vi "test Datatype Conversion.vi"(8 "error in (no error)":errorcluster, 11 "TestCase in":refnum<class "SLSC EDS Unit Tests.lvclass">) -> (0 "error out":errorcluster, 3 "TestCase out":refnum<class "SLSC EDS Unit Tests.lvclass">)   [LabVIEW 2015, in "SLSC EDS Unit Tests.lvclass"]
uses:
  SLSC EDS Unit Tests.lvclass
  <vilib>/Utility/Data Type/Type Definitions/Data Type.ctl
  <vilib>/addons/_JKI Toolkits/VI Tester/TestCase.llb/TestCase.lvclass
  <vilib>/Utility/Data Type/NI_Data Type.lvlib
  SLSC UI API/SLSC Tree Control.lvlib
panel:
  out "Pass?":bool
  out "U64":u64
  out "I32":i32
  out "I8":i8
  out "I64":i64
  out "Reset Variant Check":bool[](array[boolean])
  out "Reset = Value?":bool[](array[boolean])
  out "Value Variant Check":bool[](array[boolean])
  out "String Comparison":bool[](array[boolean])
  out "NewVal":variant
  out "Value 2 (DBL)":dbl format="%#_16f"
  out "Value":variant
  out "string data value":string
  out "Type":T1
  out "Value (DBL)":dbl format="%#_16f"
  out "U64 2":u64
  out "Numeric":i32
  in  "Ring":u16(ring)
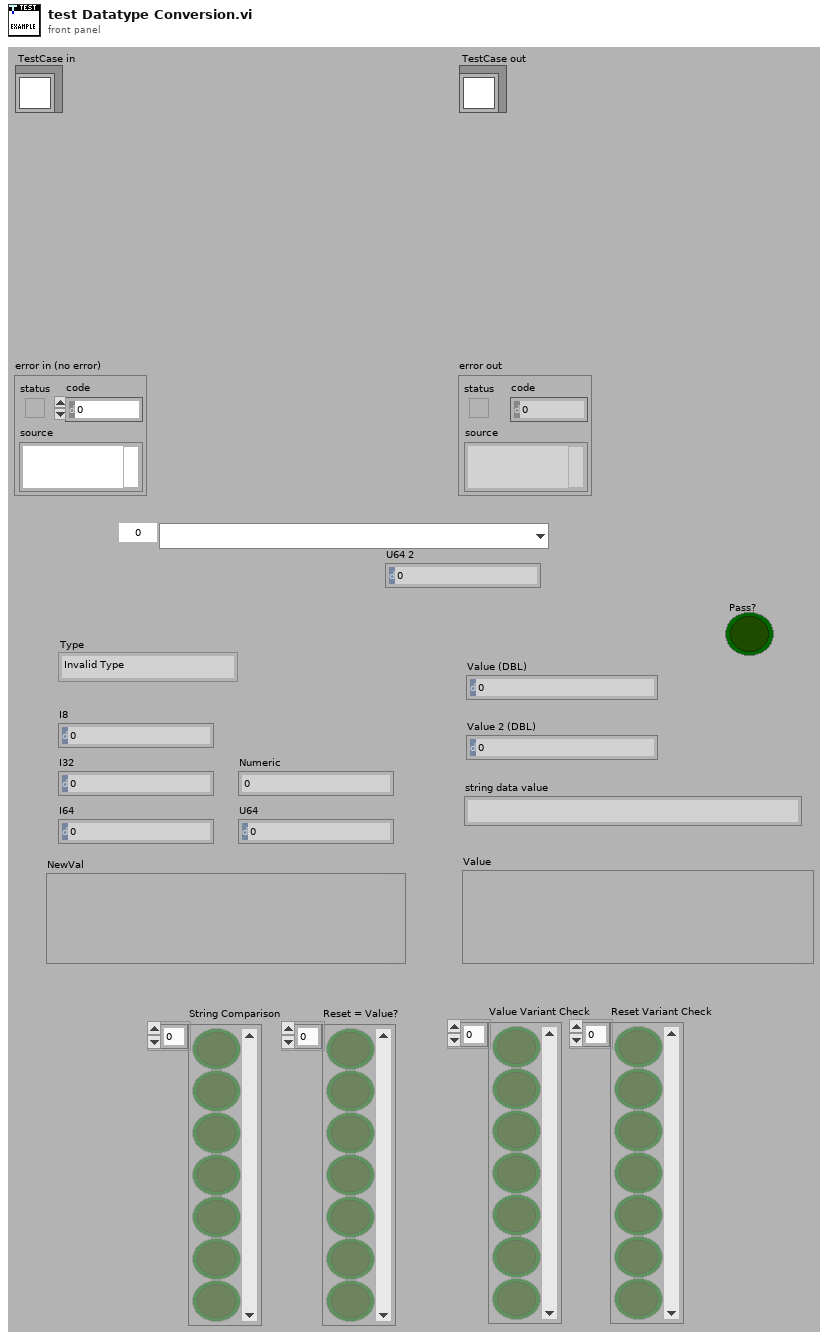
[diagram p1: front panel]
types:
  T1 = typedef "NI_Data Type.lvlib/Data Type.ctl" = enum8{"Invalid Type", "Void", "I8", "I16", "I32", "I64", "U8", "U16", "U32", "U64", "Single Float", "Double Float", "Extended Float", "Single Complex", "Double Complex", "Extended Complex", "Enum U8", "Enum U16", "Enum U32", "Enum U64", "Single Float With Unit", "Double Float With Unit", "Extended Float With Unit", "Single Complex with Unit", "Double Complex with Unit", "Extended Complex with Unit", "Boolean", "String", "Path", "Picture", "Tag", "Array", "Cluster", "Variant", "LV Variant", "Waveform", "Timestamp", "Digital Waveform", "Digital Data", "ExpressData", "Refnum", "External Data", "VI", "Poly VI", "LabVIEW Class Instance", "Fixed Point"}
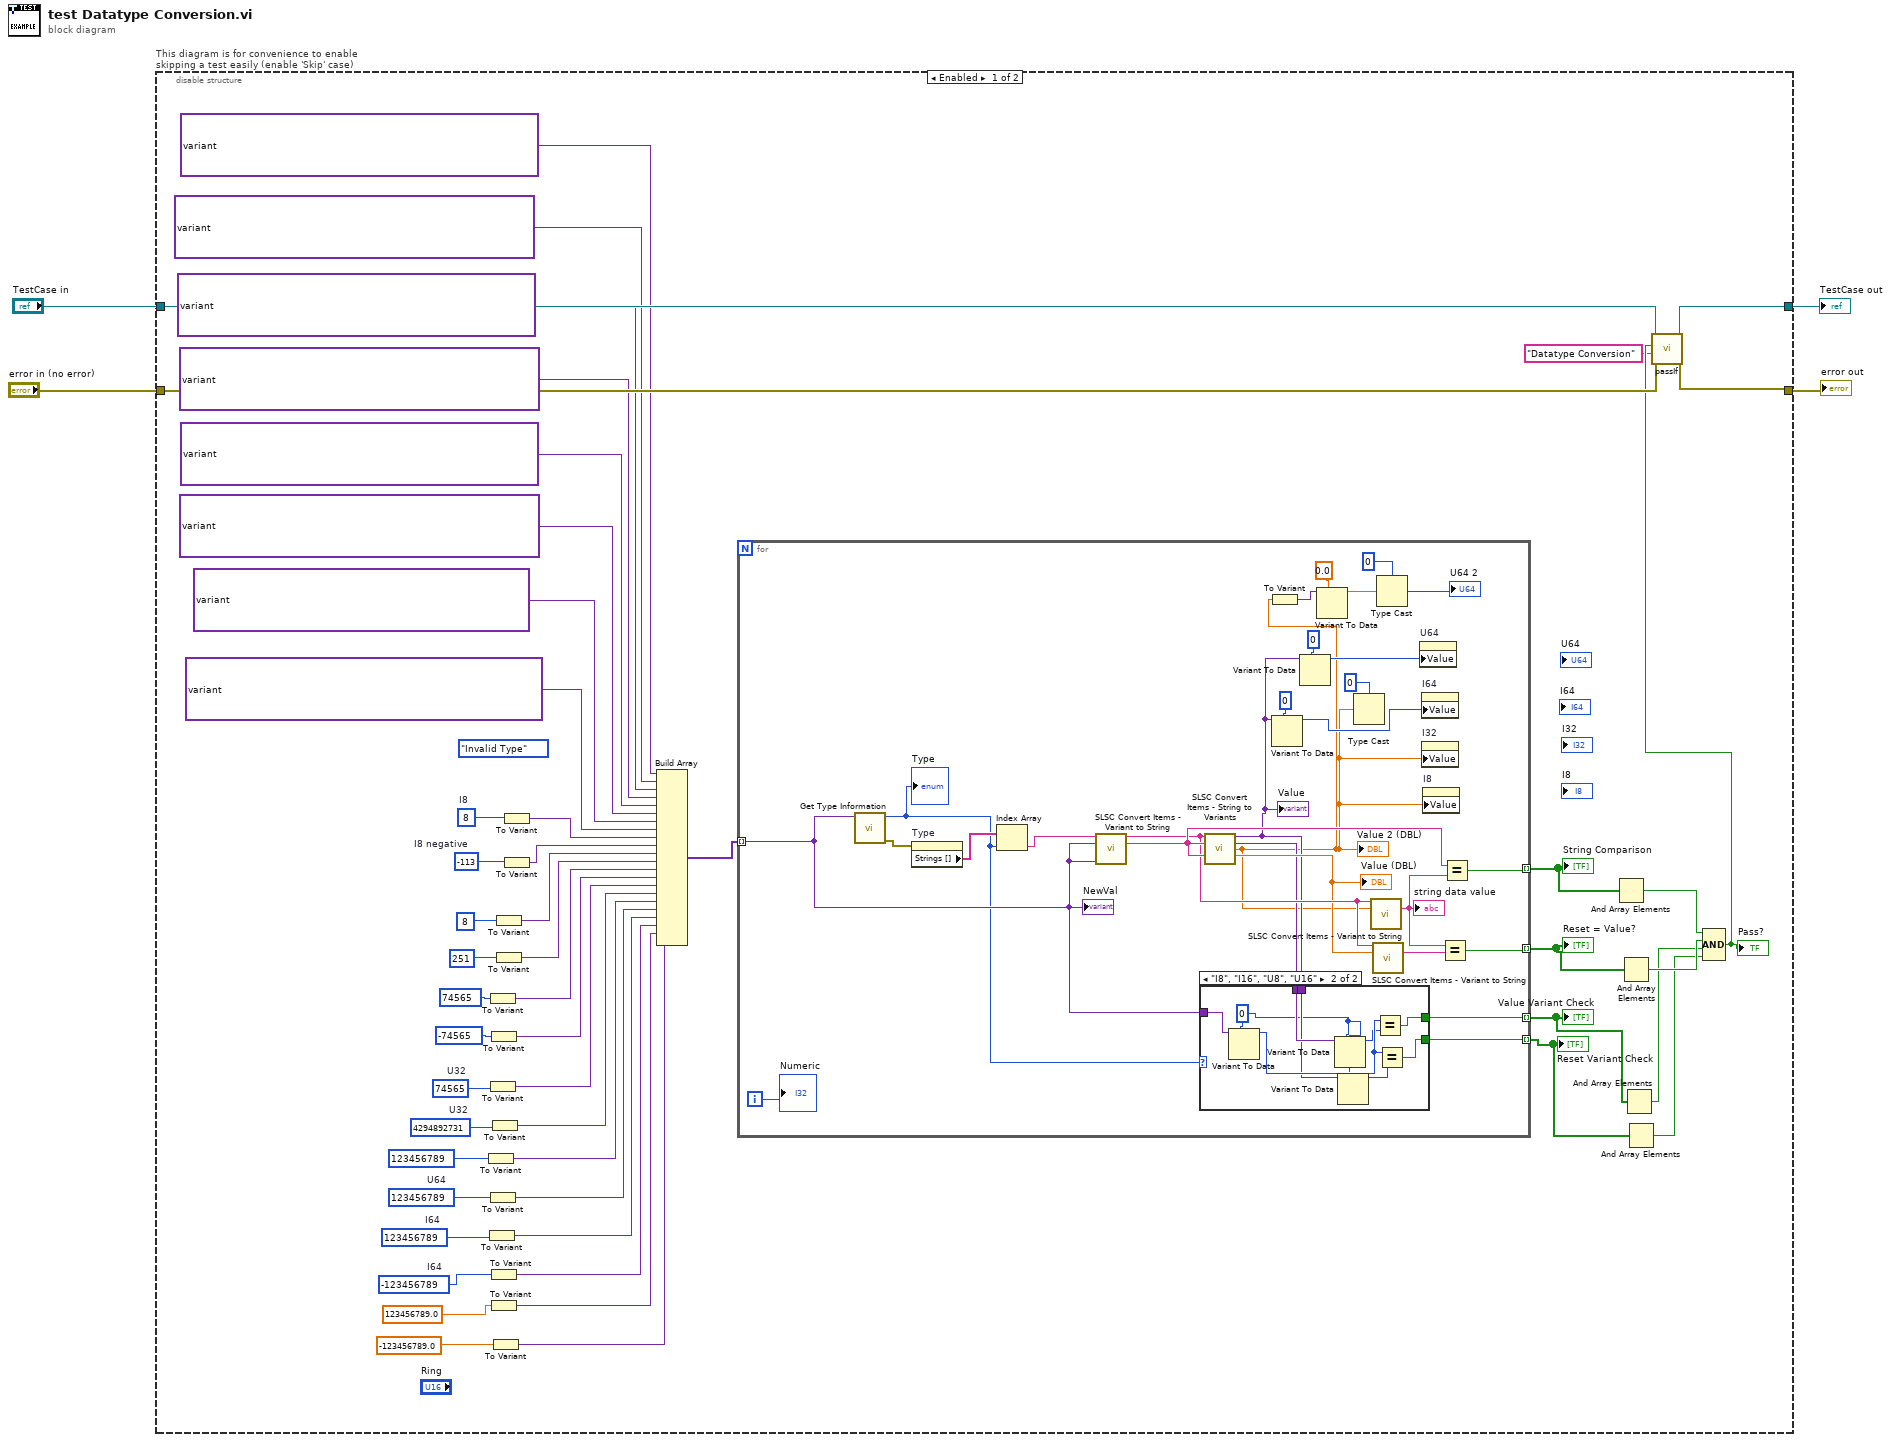
[diagram p0: block diagram]
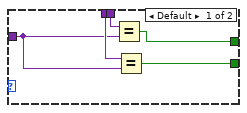
[diagram p2: hidden frame]
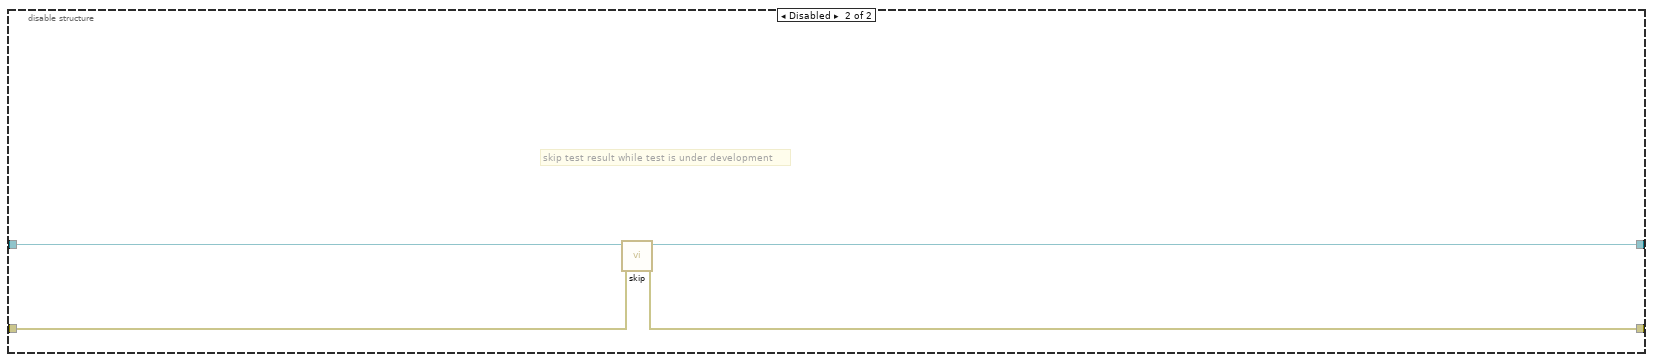
[diagram p3: hidden frame]
diagram:
  n1 = disable-structure "This diagram is for convenience to enable skipping a test easily (enable 'Skip' case)" shown="Enabled" {
    disable-tunnel: "TestCase in" -> [w55 w101]
    disable-tunnel: [w54 w99] -> w1
    disable-tunnel: [w53 w100] -> w3
    disable-tunnel: "error in (no error)" -> [w52 w98]
    frame Enabled {
      w34 = i64 -123456789  # I64
      w36 = u64 123456789  # U64
      w33 = i64 123456789  # I64
      w37 = u32 4294892731  # U32
      w38 = u32 74565  # U32
      (unwired) Data_Type."Invalid Type" ("Type")
      w50 = i8 -113  # I8 negative
      w51 = i8 8  # I8
      n2 = To Variant(anything=u64 123456789 ("U64")) -> (Variant=w30:variant)
      n3 = To Variant(anything=w33) -> (Variant=w28:variant)
      n4 = To Variant(anything=74565 ("I32")) -> (Variant=w41:variant)
      n5 = To Variant(anything=w38) -> (Variant=w32:variant)
      n6 = To Variant(anything=w36) -> (Variant=w29:variant)
      n7 = To Variant(anything=-74565 ("I32")) -> (Variant=w39:variant)
      n8 = To Variant(anything=w34) -> (Variant=w27:variant)
      n9 = To Variant(anything=123456789.0 ("DBL")) -> (Variant=w24:variant)
      n10 = To Variant(anything=w37) -> (Variant=w31:variant)
      n11 = To Variant(anything=-123456789.0 ("DBL")) -> (Variant=w23:variant)
      n12 = To Variant(anything=u8 8 ("U8")) -> (Variant=w45:variant)
      n13 = To Variant(anything=u8 251 ("U8")) -> (Variant=w43:variant)
      n14 = To Variant(anything=w51) -> (Variant=w49:variant)
      n15 = To Variant(anything=w50) -> (Variant=w48:variant)
      n16 = Build Array(variant(i32 -15) ("variant"), variant(u32 241) ("variant"), variant(i32 -3343) ("variant"), variant(u32 62193) ("variant"), variant(i32 -185339151) ("variant"), variant(u32 4109628145) ("variant"), variant(i64 -506664896818842895) ("variant"), variant(u64 17940079176890708721) ("variant"), w49, w48, w45, w43, w41, w39, w32, w31, w30, w29, w28, w27, w24, w23) -> (w47:variant[])
      n17 = for {
        tunnel: w47 -> [w71] mode=indexing
        tunnel: [w75] -> w14 mode=indexing
        tunnel: [w74] -> w13 mode=indexing
        tunnel: [w73] -> w12 mode=indexing
        tunnel: [w70] -> w11 mode=indexing
        i -> [w56]
        n18 = call <vilib>:"Get Type Information.vi"("Variant"=w71) -> ("error out"=w83:errorcluster, "Type"=w64:T1)  [unwired: 6 in, 3 out]
        "Type" <- w64
        n19 = property on="Type" class="Enum (strict)"(error in=w83) -> ("Strings []"=w82:string[])  [unwired: 1 in, 2 out]
        n20 = Index Array(array=w82, index=w64) -> (element=w81:string)
        n21 = call "SLSC Convert Items - Variant to String.vi"("Datatype"=w81, "value"=w71, "reset value"=w71) -> ("Output data type"=w79:string, "string data value"=w80:string)  [unwired: 6 in, 5 out]
        n22 = call "SLSC Convert Items - String to Variants.vi"("Datatype"=w79, "Value"=w80, "Reset Value"=w80) -> ("Value"=w61:variant, "Reset Value"=w72:variant, "Value (DBL)"=w58:dbl, "Reset Value (DBL)"=w78:dbl)  [unwired: 9 in]
        "Value 2 (DBL)" <- w58
        "Value" <- w61
        "Value (DBL)" <- w78
        n23 = case shown="\"I8\", \"I16\", \"U8\", \"U16\"" w64 {
          tunnel: [w88 w93] -> w73
          tunnel: w72 -> [w87 w96]
          tunnel: w71 -> [w86 w97]
          tunnel: [w85 w91] -> w70
          tunnel: w61 -> [w84 w92]
          frame Default {
            n24 = Equal?(x=w84, y=w86) -> (x = y?=w88:bool)
            n25 = Equal?(x=w87, y=w86) -> (x = y?=w85:bool)
          }
          frame "I8", "I16", "U8", "U16" {
            w89 = i64 0
            n26 = Variant To Data(type=w89, Variant=w97) -> (data=w95:i64)  [unwired: 1 in, 1 out]
            n27 = Variant To Data(type=w89, Variant=w96) -> (data=w94:i64)  [unwired: 1 in, 1 out]
            n28 = Variant To Data(type=w89, Variant=w92) -> (data=w90:i64)  [unwired: 1 in, 1 out]
            n29 = Equal?(x=w95, y=w94) -> (x = y?=w93:bool)
            n30 = Equal?(x=w95, y=w90) -> (x = y?=w91:bool)
          }
        }
        n31 = To Variant(anything=w58) -> (Variant=w57:variant)
        n32 = Variant To Data(type=i64 0, Variant=w61) -> (data=w67:i64)  [unwired: 1 in, 1 out]
        n33 = Variant To Data(type=u64 0, Variant=w61) -> (data=w65:u64)  [unwired: 1 in, 1 out]
        n34 = Variant To Data(type=0.0, Variant=w57) -> (data=w62:dbl)  [unwired: 1 in, 1 out]
        n35 = Type Cast(type=i64 0 ("I64"), x=w58) -> ()  [unwired: 1 out]
        n36 = call "SLSC Convert Items - Variant to String.vi"("Datatype"=w79, "value"=w58) -> ("string data value"=w76:string)  [unwired: 7 in, 6 out]
        "string data value" <- w76
        n37 = call "SLSC Convert Items - Variant to String.vi"("Datatype"=w79, "value"=w78) -> ("string data value"=w77:string)  [unwired: 7 in, 6 out]
        n38 = Type Cast(type=i64 0, x=w62) -> (*(type *) &x=→"U64 2":i64)
        n39 = property on="U64" class="DigNum (strict)"("Value"=w65) -> ()  [unwired: 2 in, 2 out]
        n40 = property on="I64" class="DigNum (strict)"("Value"=w67) -> ()  [unwired: 2 in, 2 out]
        n41 = property on="I32" class="DigNum (strict)"("Value"=w58) -> ()  [unwired: 2 in, 2 out]
        n42 = property on="I8" class="DigNum (strict)"("Value"=w58) -> ()  [unwired: 2 in, 2 out]
        n43 = Equal?(x=w76, y=w77) -> (x = y?=w74:bool)
        n44 = Equal?(x=w80, y=w76) -> (x = y?=w75:bool)
        "NewVal" <- w71
        "Numeric" <- w56
      }
      "String Comparison" <- w14
      "Value Variant Check" <- w12
      "Reset = Value?" <- w13
      "Reset Variant Check" <- w11
      n45 = And Array Elements(Boolean array=w14) -> (logical AND=w10:bool)
      n46 = And Array Elements(Boolean array=w13) -> (logical AND=w9:bool)
      n47 = And Array Elements(Boolean array=w12) -> (logical AND=w8:bool)
      n48 = And Array Elements(Boolean array=w11) -> (logical AND=w7:bool)
      n49 = Compound Arithmetic op=AND(w10, w9, w8, w7) -> (w6:bool)
      "Pass?" <- w6
      n50 = call-dynamic "passIf.vi"("error in (no error)"=w52, "message (\"\")"="Datatype Conversion" ("message (\"\")"), "pass"=w6, "TestCase in"=w55) -> ("error out"=w53:errorcluster, "TestCase out"=w54:refnum<class "SLSC EDS Unit Tests.lvclass">)  [unwired: 6 in]
    }
    frame Disabled {
      # "skip test result while test is under development"
      n51 = call <vilib>:"skip.vi"("error in (no error)"=w98, "TestCase in"=w101) -> ("error out"=w100:errorcluster, "TestCase out"=w99:refnum<class "SLSC EDS Unit Tests.lvclass">)  [unwired: 8 in]
    }
  }
  "error out" <- w3
  "TestCase out" <- w1
